vi "Read uStringManipulation.vi"(8 "error in (no error)":errorcluster, 11 "uPolicy in":refnum<class "uPolicy.lvclass">) -> (0 "error out":errorcluster, 2 "uStringManipulation.lvlib:uStringManipulation.lvclass":refnum<class "uStringManipulation.lvclass">, 3 "uPolicy out":refnum<class "uPolicy.lvclass">)   [LabVIEW 2023, in "uLib.lvlib" / "uPolicy.lvclass"]
uses:
  uPolicy.lvclass
  uStringManipulation/uStringManipulation/uStringManipulation.lvclass
  uPolicy.lvclass/uPolicy.ctl
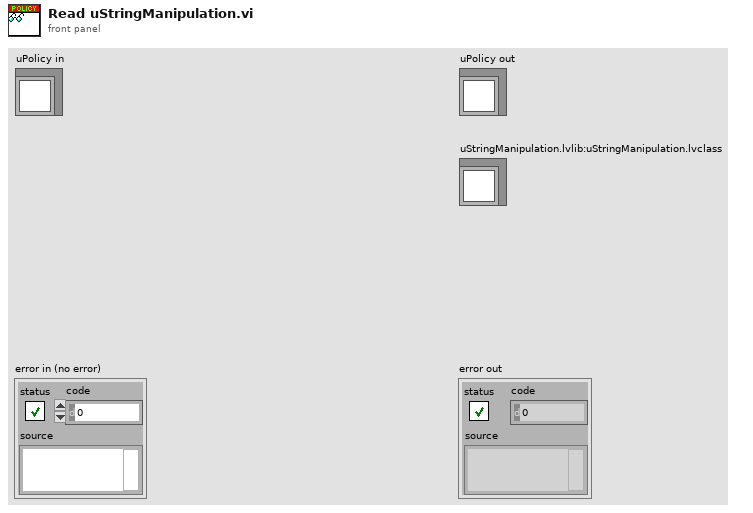
[diagram p1: front panel]
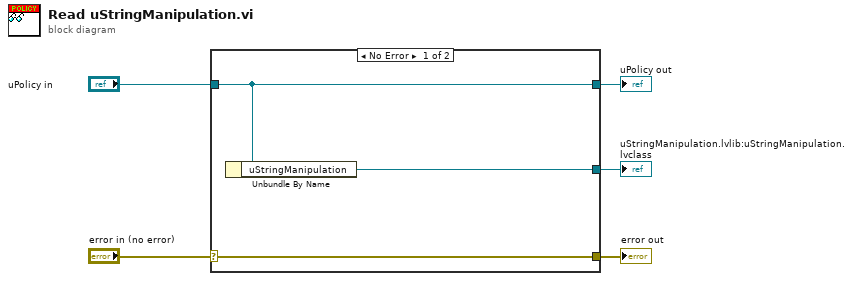
[diagram p0: block diagram]
diagram:
  n1 = case shown="No Error" "error in (no error)" {
    selector: "error in (no error)" -> [w8 w9]
    tunnel: [w8 w9] -> w4
    tunnel: [w7 w10] -> w2
    tunnel: "uPolicy in" -> [w7 w10]
    tunnel: [w6 _] -> w1
    frame No Error {
      n2 = Unbundle By Name(w7) -> ("uStringManipulation"=w6:refnum<class "uStringManipulation.lvclass">)
    }
    frame Error {
    }
  }
  "error out" <- w4
  "uPolicy out" <- w2
  "uStringManipulation.lvlib:uStringManipulation.lvclass" <- w1
